vi "Get Section Data.vi"(8 "error in":errorcluster, 11 "Section in":refnum<class "Section.lvclass">) -> (0 "error out":errorcluster, 2 "Section Data":T1, 3 "Section out":refnum<class "Section.lvclass">)   [LabVIEW 2024, in "Parser.lvlib" / "Section.lvclass"]
uses:
  Section.lvclass
  Section.lvclass/Section.ctl
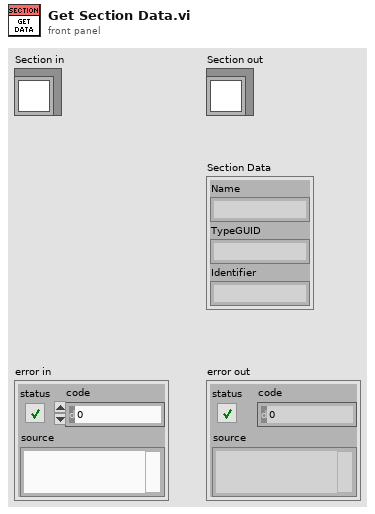
[diagram p1: front panel]
types:
  T1 = cluster{"Name":string, "TypeGUID":string, "Identifier":string}
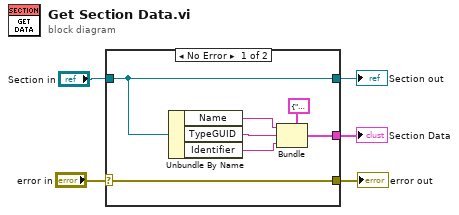
[diagram p0: block diagram]
diagram:
  n1 = case shown="No Error" "error in" {
    selector: "error in" -> [w12 w14]
    tunnel: [w11 _] -> w3
    tunnel: "Section in" -> [w6 w13]
    tunnel: [w12 w14] -> w4
    tunnel: [w6 w13] -> w1
    frame No Error {
      n2 = Unbundle By Name(w6) -> ("Name"=w9:string, "TypeGUID"=w8:string, "Identifier"=w7:string)
      n3 = Bundle(cluster=T1 {"Name"="", "TypeGUID"="", "Identifier"=""}, "Name"=w9, "TypeGUID"=w8, "Identifier"=w7) -> (w11:T1)
    }
    frame Error {
    }
  }
  "error out" <- w4
  "Section Data" <- w3
  "Section out" <- w1
